vi "launch vi server handler.vi"(8 "error in":errorcluster, 9 "command line arguments":T1, 10 "base path":path, 11 "Application in":refnum<vi>) -> (0 "error out":errorcluster)   [LabVIEW 2013]
uses:
  arguments.ctl
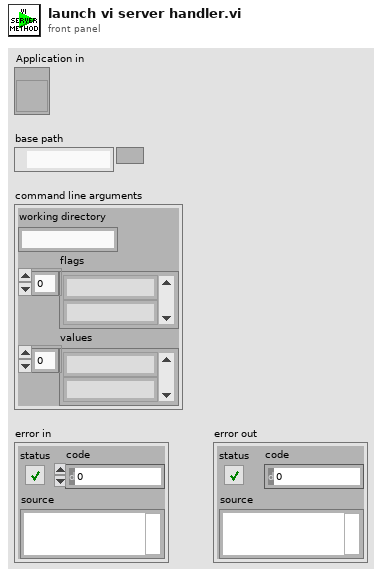
[diagram p1: front panel]
types:
  T1 = typedef "arguments.ctl" = cluster{"working directory":string, "flags":string[], "values":string[]}
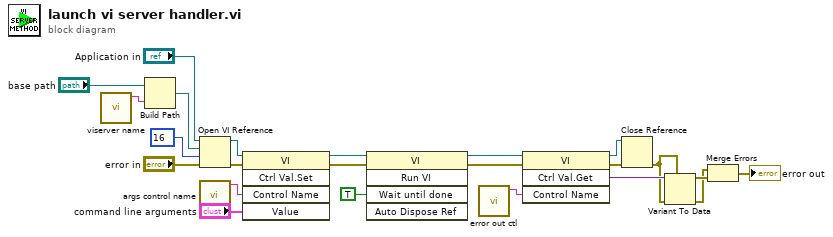
[diagram p0: block diagram]
diagram:
  n1 = call "viserver name.vi"() -> ("viserver vi name"=w23:string)  [unwired: 11 in]
  n2 = Build Path(base path="base path", name or relative path=w23) -> (appended path=w3:path)
  n3 = Open VI Reference(application reference (local)="Application in", vi path=w3, options=16, error in (no error)="error in") -> (vi reference=w6:refnum<vi>, error out=w5:errorcluster)  [unwired: 2 in]
  n4 = call "args control name.vi"() -> ("args control name"=w10:string)  [unwired: 11 in]
  n5 = invoke class="VI" method="Ctrl Val.Set"(reference=w6, error in=w5, "Control Name"=w10, "Value"="command line arguments") -> (reference out=w7:refnum<vi>, error out=w8:errorcluster)  [unwired: 1 in, 3 out]
  n6 = invoke class="VI" method="Run VI"(reference=w7, error in=w8, "Wait until done"=TRUE ("Wait Until Done")) -> (reference out=w12:refnum<vi>, error out=w15:errorcluster)  [unwired: 2 in, 3 out]
  n7 = call "error out ctl.vi"() -> ("error out control"=w17:string)  [unwired: 11 in]
  n8 = invoke class="VI" method="Ctrl Val.Get"(reference=w12, error in=w15, "Control Name"=w17) -> (reference out=w14:refnum<vi>, error out=w16:errorcluster, "Get Control Value Variant"=w20:variant)  [unwired: 1 in, 1 out]
  n9 = Close Reference(reference=w14, error in (no error)=w16) -> (error out=w19:errorcluster)
  n10 = Variant To Data(error in=w19, type=w19, Variant=w20) -> (data=w22:errorcluster, error out=w18:errorcluster)
  n11 = Merge Errors(w18, w22) -> (→"error out":errorcluster)
